vi "SWS_LicenseInfo.vi"() -> ()   [LabVIEW 2014]
panel:
  out "concatenated string":string
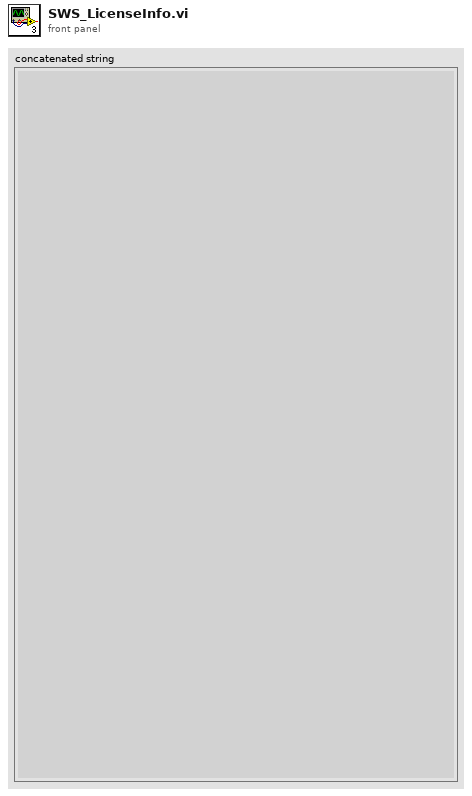
[diagram p1: front panel]
types:
  T1 = typedef "Registry refnum.ctl" = refnum<k1>
  T2 = cluster{"numSubKeys":i32, "maxSubKeyLen":i32, "maxSubKeyClassLen":i32}
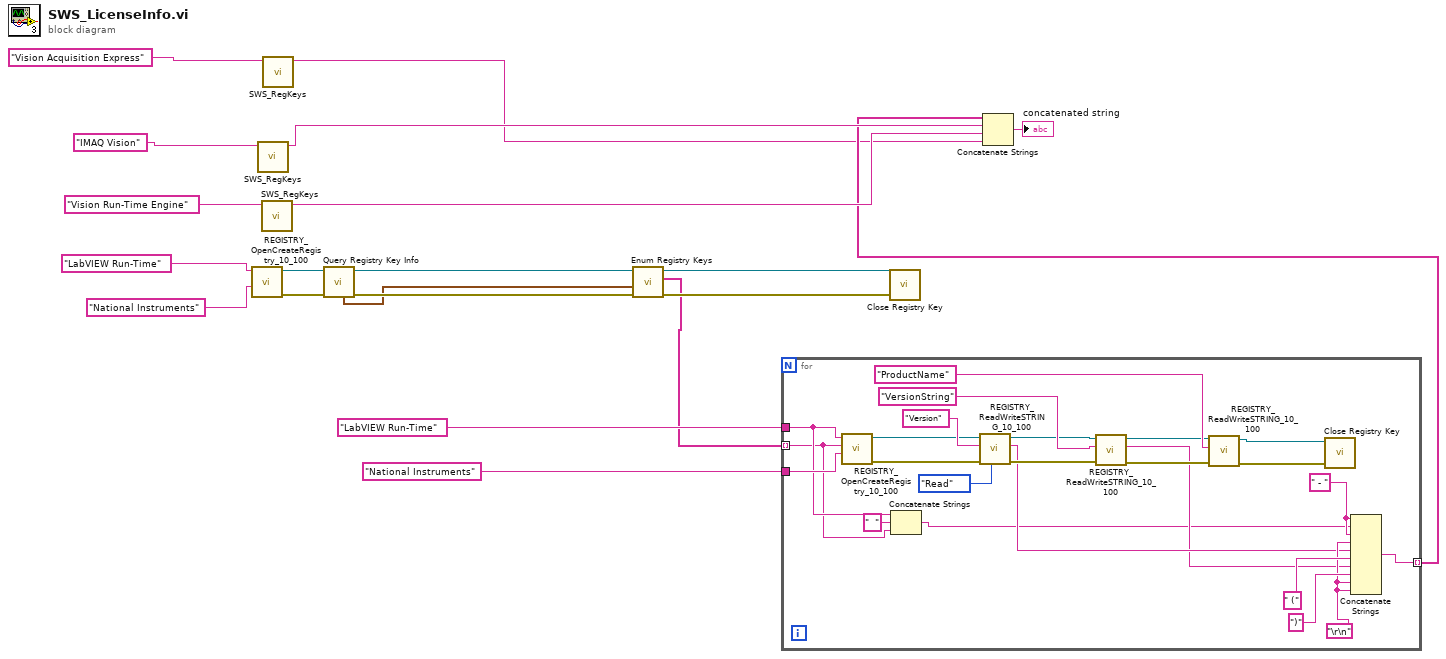
[diagram p0: block diagram]
diagram:
  n1 = call <vilib>:"REGISTRY_OpenCreateRegistry_10_100.vi"("Section (SoftWire Systems)"="National Instruments" ("Application Name"), "Application Name"="LabVIEW Run-Time") -> ("error out"=w10:errorcluster, "refnum out"=w11:T1)  [unwired: 4 in]
  n2 = call "SWS_RegKeys.vi"("Application Name"="IMAQ Vision") -> ("NI Registry Info"=w18:string)  [unwired: 10 in]
  n3 = call "SWS_RegKeys.vi"("Application Name"="Vision Run-Time Engine") -> ("NI Registry Info"=w17:string)  [unwired: 10 in]
  n4 = call "SWS_RegKeys.vi"("Application Name"="Vision Acquisition Express") -> ("NI Registry Info"=w1:string)  [unwired: 10 in]
  n5 = call <vilib>:"Query Registry Key Info.vi"("error in (no error)"=w10, "refnum"=w11) -> ("error out"=w9:errorcluster, "refnum out"=w8:T1, "subkey info"=w7:T2)  [unwired: 5 in, 2 out]
  n6 = call <vilib>:"Enum Registry Keys.vi"("error in (no error)"=w9, "subkey info"=w7, "refnum"=w8) -> ("error out"=w12:errorcluster, "subkeys"=w4:string[], "refnum out"=w13:T1)  [unwired: 6 in]
  n7 = for {
    tunnel: "LabVIEW Run-Time" ("Application Name") -> [w24]
    tunnel: "National Instruments" ("Application Name") -> [w44]
    tunnel: w4 -> [w22] mode=indexing
    tunnel: [w25] -> w2 mode=indexing
    w28 = "\r\n"
    w30 = " - " ("string")
    n8 = call <vilib>:"REGISTRY_OpenCreateRegistry_10_100.vi"("Section (SoftWire Systems)"=w44, "Key Group"=w22, "Application Name"=w24) -> ("error out"=w35:errorcluster, "refnum out"=w34:T1)  [unwired: 3 in]
    n9 = Concatenate Strings(w24, "  " ("string"), w22) -> (w21:string)
    n10 = call <vilib>:"REGISTRY_ReadWriteSTRING_10_100.vi"("Mode"=enum16{"Read", "Write"}."Read", "error in (no error)"=w35, "Key Name"="Version" ("Application Name"), "refnum in"=w34) -> ("error out"=w38:errorcluster, "Key Data Out"=w27:string, "refnum out"=w40:T1)  [unwired: 5 in]
    n11 = call <vilib>:"REGISTRY_ReadWriteSTRING_10_100.vi"("error in (no error)"=w38, "Key Name"="VersionString" ("Application Name"), "refnum in"=w40) -> ("error out"=w39:errorcluster, "Key Data Out"=w26:string, "refnum out"=w41:T1)  [unwired: 6 in]
    n12 = call <vilib>:"REGISTRY_ReadWriteSTRING_10_100.vi"("error in (no error)"=w39, "Key Name"="ProductName" ("Application Name"), "refnum in"=w41) -> ("error out"=w32:errorcluster, "refnum out"=w33:T1)  [unwired: 6 in, 1 out]
    n13 = call <vilib>:"Close Registry Key.vi"("error in (no error)"=w32, "refnum"=w33) -> ()  [unwired: 5 in, 1 out]
    n14 = Concatenate Strings(w30, w21, w30, w28, w27, " (", w26, ")", w28, w28) -> (w25:string)
  }
  n15 = call <vilib>:"Close Registry Key.vi"("error in (no error)"=w12, "refnum"=w13) -> ()  [unwired: 5 in, 1 out]
  n16 = Concatenate Strings(w2, w18, w17, w1) -> (→"concatenated string":string)
